vi "字符串 与路径 数据 - 2.vi"() -> ()   [LabVIEW 2023]
panel:
  out "Boolean array":bool[](array[boolean])
  out "reversed array":bool[](array[boolean])
  in  "String":string
  # "字符串 与路径 数据 - 2"
  # "不太明白 18 进制转换为 布尔数组 为啥是32 个布尔量\n但是 好似不太重要。先略过，以后再说。"
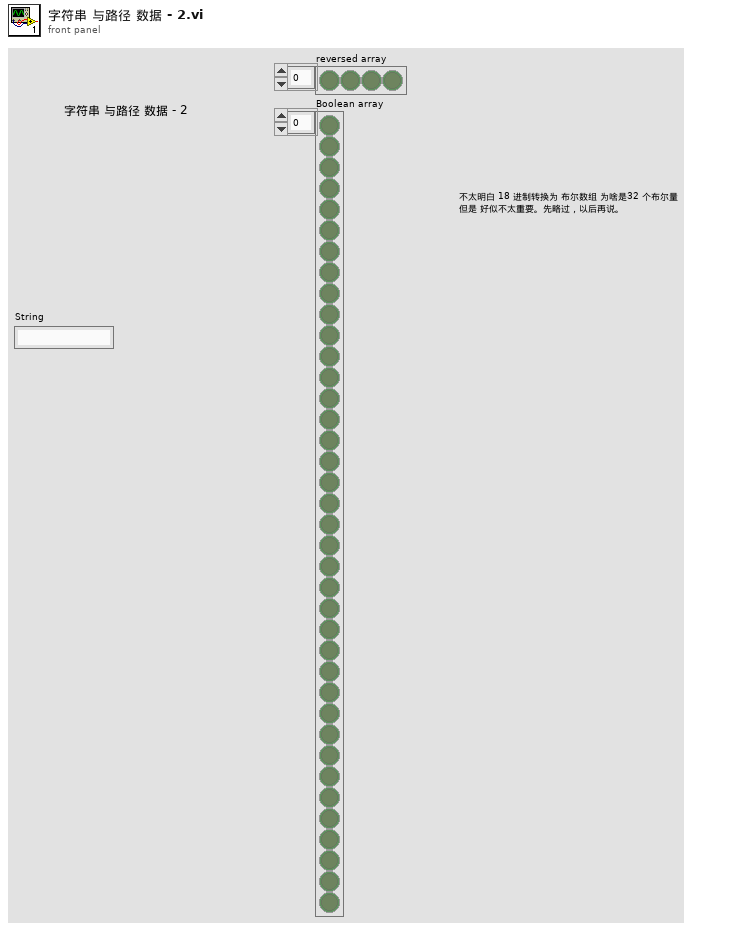
[diagram p1: front panel]
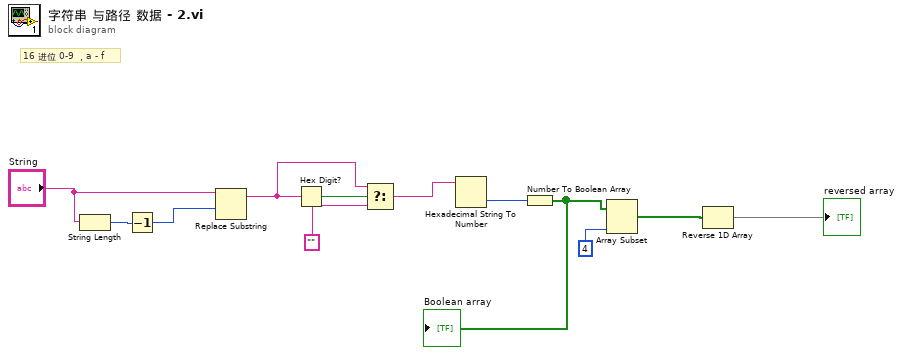
[diagram p0: block diagram]
diagram:
  # "16 进位 0-9 ，a - f"
  n1 = String Length(string="String") -> (length=w12:i32)
  n2 = Decrement(x=w12) -> (x-1=w11:i32)
  n3 = Replace Substring(3:w11, 5:"String") -> (1:w8:string)  [unwired: 2 in, 1 out]
  n4 = Hex Digit?(1:w8) -> (0:w9:bool)
  n5 = Select(t=w8, s=w9, f="") -> (s? t:f=w6:string)
  n6 = Hexadecimal String To Number(string=w6) -> (number=w5:u32)  [unwired: 2 in, 1 out]
  n7 = Number To Boolean Array(number=w5) -> (Boolean array=w1:bool[])
  "Boolean array" <- w1
  n8 = Array Subset "Array Subset"(array=w1, length=4) -> (w3:bool[])  [unwired: 1 in]
  n9 = Reverse 1D Array(array=w3) -> (reversed array=→"reversed array":bool[])
